vi "StellarNet_Get_Spectra_timed.vi"(0 "Integration Time (ms)":i32=80 caption="Inter scan delay ms", 5 "Number of Scans to Average":i32=1 min=1 max=10000 step=1, 7 "Digitizer Clock Rate Setting":i32=3 min=1 max=3, 9 "Optical Smoothing Level":i32 min=0 max=4 step=1) -> (4 "Spectrum":cluster{"Wavelengths":dbl[], "buffer out":sgl[]}(graph), 6 "output param":i32, 10 "Critical Error":bool)   [LabVIEW 2014]
uses:
  <vilib>/Utility/file.llb/Write To Spreadsheet File (string).vi
  <vilib>/Utility/file.llb/Write To Spreadsheet File (DBL).vi
panel:
  in  "Seconds between \nspectra":dbl caption="Time Target (s)"
  in  "stop":bool
  in  "?":path=path "C:/Users/User/Desktop/Chamber Data/perovskites/2015-08-04 spectra"
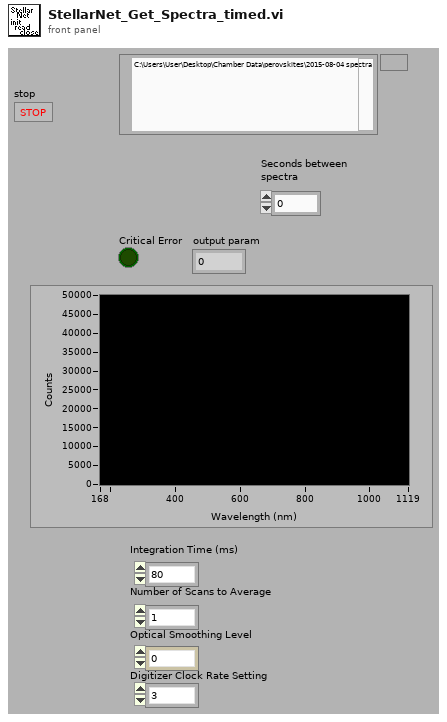
[diagram p1: front panel]
types:
  T1 = cluster{"Coefficients":ext[], "Wavelengths":dbl[]}[]
  T2 = cluster{"Integration Time (ms)":i32, "Number of Scans to Average":i32, "Optical Smoothing Level":i32, "Digitizer Clock Rate Setting":i32, "Temp  Compensation ":bool}[]
  T3 = cluster{"Integration Time (ms)":i32, "Number of Scans to Average":i32, "Optical Smoothing Level":i32, "Digitizer Clock Rate Setting":i32, "Temp  Compensation ":bool}
  T4 = cluster{"Coefficients":ext[], "Wavelengths":dbl[]}
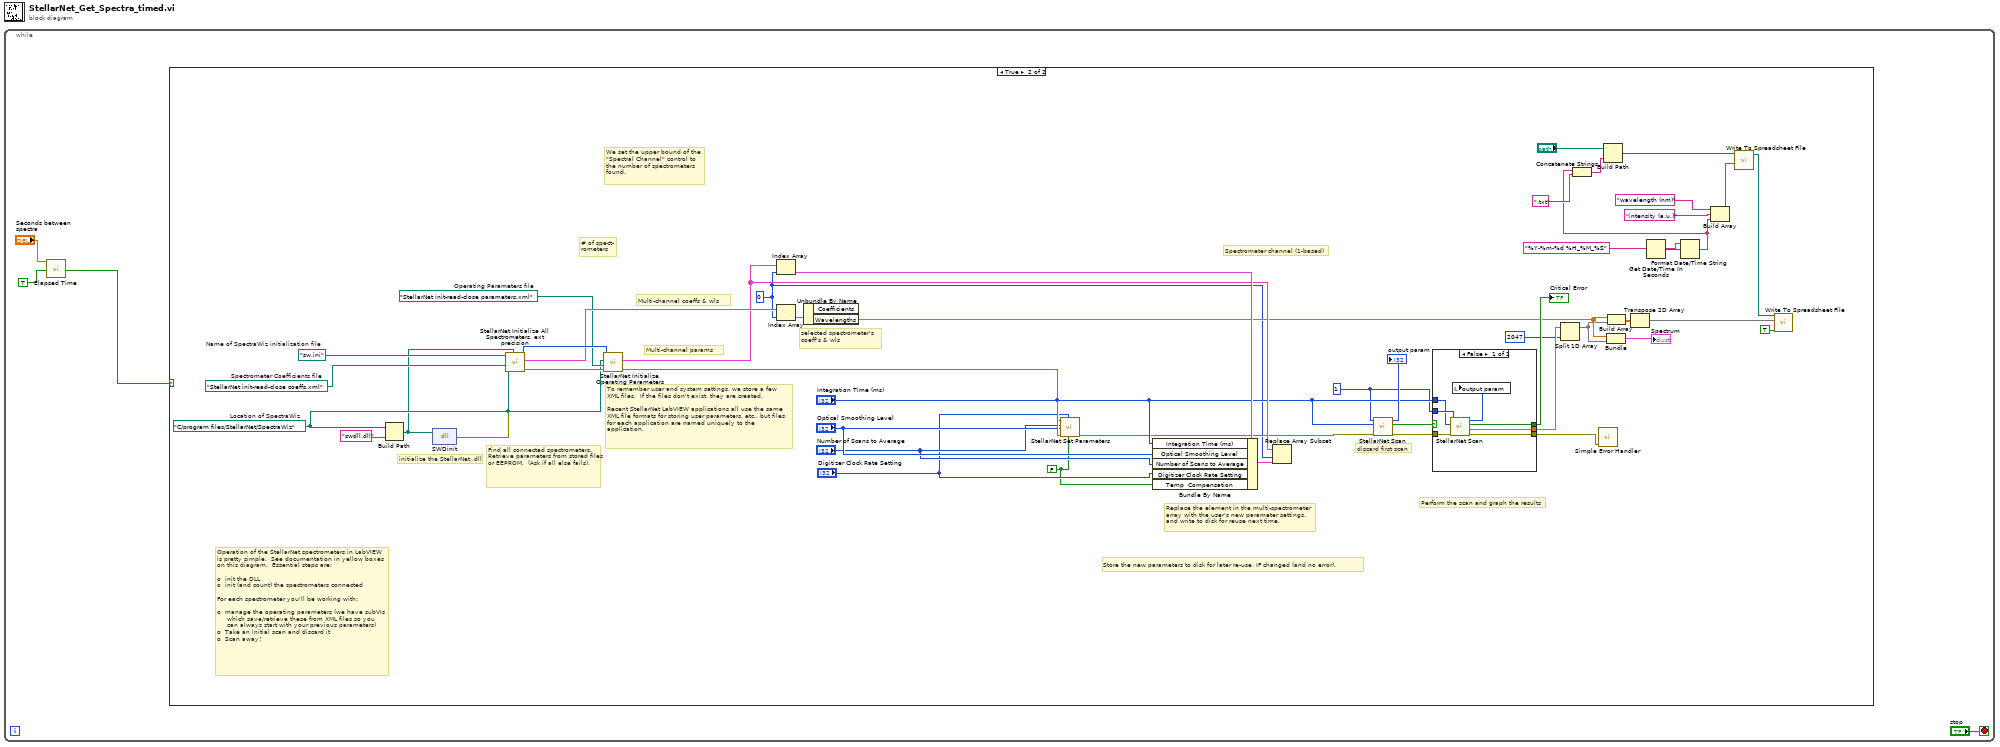
[diagram p0: block diagram]
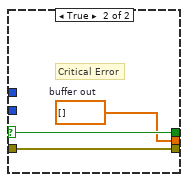
[diagram p3: hidden frame]
diagram:
  n1 = while {
    stop <- "stop" stop-if-true
    n2 = call "Elapsed Time"("Time Target (s)"="Seconds between \nspectra", "Auto Reset"=TRUE) -> ("Time has Elapsed"=w2:bool)  [unwired: 10 in, 7 out]
    n3 = case shown="True" w2 {
      frame False {
      }
      frame True {
        w19 = 0 ("Spectral Channel")
        w21 = 1 ("Spectral Channel")
        w25 = FALSE ("Temp  Compensation")
        w33 = path "C:/program files/StellarNet/SpectraWiz"  # Location of SpectraWiz
        w43 = path "sw.ini"  # Name of SpectraWiz initialization file
        w35 = path "StellarNet init-read-close parameters.xml"  # Operating Parameters file
        w44 = path "StellarNet init-read-close coeffs.xml"  # Spectrometer Coefficients file
        # "Replace the element in the multi-spectrometer\narray with the user's new parameter settings,\nand write to disk for reuse next time."
        # "Operation of the StellarNet spectrometers in LabVIEW\nis pretty simple.  See documentation in yellow boxes\non this diagram.  Essential steps are:\n\no  init the DLL\no  init (and count) the spectrometers connected\n\nFor each spectrometer you'll be working with:\n\no  manage the operating parameters (we have subVIs\n     which save/retrieve these from XML files so you\n     can always start with your previous parameters)\no  Take an initial scan and discard it\no  Scan away!"
        # "initialize the StellarNet .dll"
        # "Spectrometer channel (1-based)"
        # "Perform the scan and graph the results"
        # "We set the upper bound of the\n\"Spectral Channel\" control to \nthe number of spectrometers \nfound."
        # "To remember user and system settings, we store a few \nXML files.  If the files don't exist, they are created.\n\nRecent StellarNet LabVIEW applications all use the same\nXML file formats for storing user parameters, etc., but files\nfor each application are named uniquely to the \napplication."
        # "Store the new parameters to disk for later re-use, IF changed (and no error)."
        # "Find all connected spectrometers.  Retrieve parameters from stored files or EEPROM.  (Ask if all else fails)."
        # "selected spectrometer's\ncoeff's & wls"
        # "Multi-channel coeffs & wls"
        # "# of spect-\nrometers"
        # "Multi-channel params"
        # "discard first scan"
        n4 = Build Path(base path=w33, name or relative path="swdll.dll") -> (appended path=w31:path)
        n5 = dll-call lib="C:/Program Files/StellarNet/SpectraWiz/swdll.dll" fn="SWDinit" label="init"(path in=w31) -> (error out=w32:errorcluster)  [unwired: 3 in, 1 out]
        n6 = call "StellarNet Initialize All Spectrometers, ext precision.vi"("Path of swdll.dll"=w31, "error in"=w32, "Spectrometer Coefficients file"=w44, "Location of SpectraWiz"=w33, "Name of SpectraWiz initialization file"=w43) -> ("error out"=w42:errorcluster, "Multi Channel Coeffs & WLs"=w40:T1, "Number of Channels"=w41:i32)  [unwired: 2 in, 2 out]
        n7 = call "StellarNet Initialize Operating Parameters.vi"("error in"=w42, "Spectrometer Coefficients file"=w35, "Location of SpectraWiz"=w33, "Number of Channels"=w41) -> ("error out"=w38:errorcluster, "Operating Parameters"=w36:T2)  [unwired: 6 in]
        n8 = Index Array(array=w36, index=w19) -> (element=w37:T3)
        n9 = Index Array(array=w40, index=w19) -> (element=w39:T4)
        n10 = Unbundle By Name(w39) -> ("Wavelengths"=w23:dbl[])  [unwired: 1 out]
        n11 = call "StellarNet Set Parameters.vi"("Temp  Compensation"=w25, "Digitizer Clock Rate Setting"="Digitizer Clock Rate Setting", "error in (no error)"=w38, "Optical Smoothing Level"="Optical Smoothing Level", "Number of Scans to Average"="Number of Scans to Average", "Integration Time (ms)"="Integration Time (ms)") -> ("error out"=w24:errorcluster)  [unwired: 5 in]
        n12 = Bundle By Name(cluster=w37, "Integration Time (ms)"="Integration Time (ms)", "Optical Smoothing Level"="Optical Smoothing Level", "Number of Scans to Average"="Number of Scans to Average", "Digitizer Clock Rate Setting"="Digitizer Clock Rate Setting", "Temp  Compensation"=w25) -> (w28:T3)
        n13 = Replace Array Subset(array=w36, new element=w28, index=w19) -> ()  [unwired: 1 out]
        n14 = call "StellarNet Scan.vi"("error in (no error)"=w24, "Integration Time (msec)"="Integration Time (ms)", "Spectral Channel"=w21) -> ("error out"=w49:errorcluster, "Critical Error"=w50:bool, "output param"=→"output param":i32)  [unwired: 5 in, 1 out]
        n15 = case shown="False" w50 {
          selector: w50 -> [_ w61]
          tunnel: w21 -> [w58 _]
          tunnel: [w57 w60] -> w34
          tunnel: [w55 w61] -> w47
          tunnel: w49 -> [w54 w59]
          tunnel: [w53 w59] -> w20
          tunnel: "Integration Time (ms)" -> [w52 _]
          frame False {
            n16 = call "StellarNet Scan.vi"("error in (no error)"=w54, "Integration Time (msec)"=w52, "Spectral Channel"=w58) -> ("error out"=w53:errorcluster, "buffer out"=w57:sgl[], "Critical Error"=w55:bool, "output param"=w56:i32)  [unwired: 5 in]
            n17 = local write "output param"(w56) -> ()
          }
          frame True {
            w60 = sgl[] []  # buffer out
            # "Critical Error"
          }
        }
        "Critical Error" <- w47
        n18 = Split 1D Array(array=w34, index=2047) -> (first subarray=w22:sgl[])  [unwired: 1 out]
        n19 = call <vilib>:"Simple Error Handler.vi"("error in (no error)"=w20) -> ()  [unwired: 4 in, 5 out]
        n20 = Bundle("Wavelengths"=w23, w22) -> (→"Spectrum":cluster{"Wavelengths":dbl[], sgl[]})  [unwired: 1 in]
        n21 = Build Array(w23, w22) -> (w7:dbl[][])
        n22 = Transpose 2D Array(2D array=w7) -> (transposed array=w6:dbl[][])
        n23 = Get Date/Time In Seconds() -> (seconds since 1Jan1904=w13:timestamp)
        n24 = Format Date/Time String(time format string (%c)="%Y-%m-%d %H_%M_%S", seconds (now)=w13) -> (date/time string=w8:string)  [unwired: 1 in]
        n25 = Concatenate Strings(w8, ".txt") -> (w9:string)
        n26 = Build Path(base path="?", name or relative path=w9) -> (appended path=w11:path)
        n27 = Build Array("wavelength (nm)", "intensity (a.u.)", w8) -> (w14:string[])
        n28 = call-poly <vilib>:"Write To Spreadsheet File.vi"("1D data"=w14, "file path (dialog if empty)"=w11) -> ("new file path (Not A Path if cancelled)"=w5:path)  [unwired: 6 in]
        n29 = call-poly <vilib>:"Write To Spreadsheet File.vi"("append to file? (new file:F)"=TRUE, "2D data"=w6, "file path (dialog if empty)"=w5) -> ()  [unwired: 5 in, 1 out]
      }
    }
  }
